vi "Validate_Cal_Date.vi"(10 "Calibration Limit(Days)":u32=120, 11 "Calibration File Paths":path[](array[path])=[path "C:/Users/Public/Documents/TDS Data/Rampage 5G HPA Pallet/Calibration/SigGen_plus_Cable.ini", path "C:/Users/Public/Documents/TDS Data/Rampage 5G HPA Pallet/Calibration/RF_to_UUT_HPA.ini", path "C:/Users/Public/Documents/TDS Data/Rampage 5G HPA Pallet/Calibration/RF_from_UUT_HPA.ini"]) -> (0 "Read Error?":bool, 1 "Calibration Due?":bool, 2 "found?":bool)   [LabVIEW 2025]
uses:
  <vilib>/Utility/miscctls.llb/LVDateTimeRec.ctl
  <vilib>/Utility/config.llb/Read Key (String).vi
  <vilib>/Utility/config.llb/NI_LVConfig.lvlib
panel:
  out "Current time":timestamp
  out "Calibration Date/Time":timestamp
  out "value":string
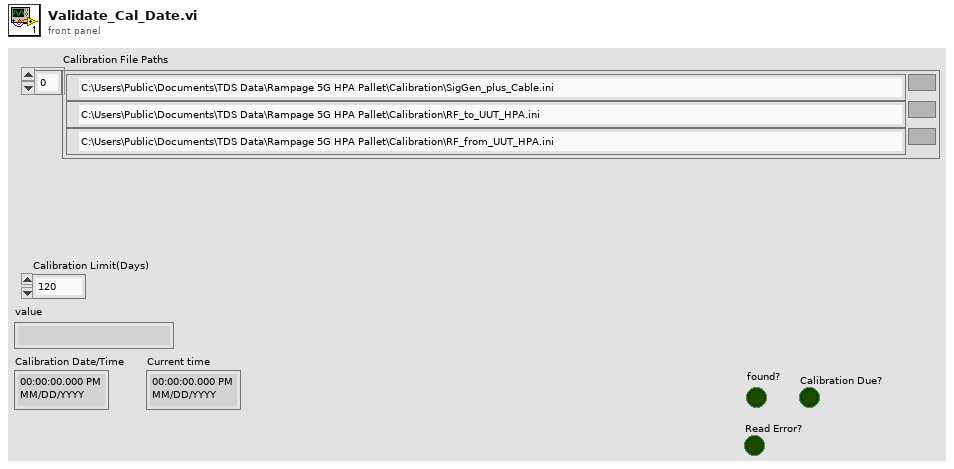
[diagram p1: front panel]
types:
  T1 = typedef "LVDateTimeRec.ctl" = cluster{"fractional second":dbl, "second":i32, "minute":i32, "hour":i32, "day of month":i32, "month":i32, "year":i32, "day of week":i32, "day of year":i32, "DST":i32}
  T2 = typedef "NI_LVConfig.lvlib/Config Data RefNum.ctl" = refnum<k1>
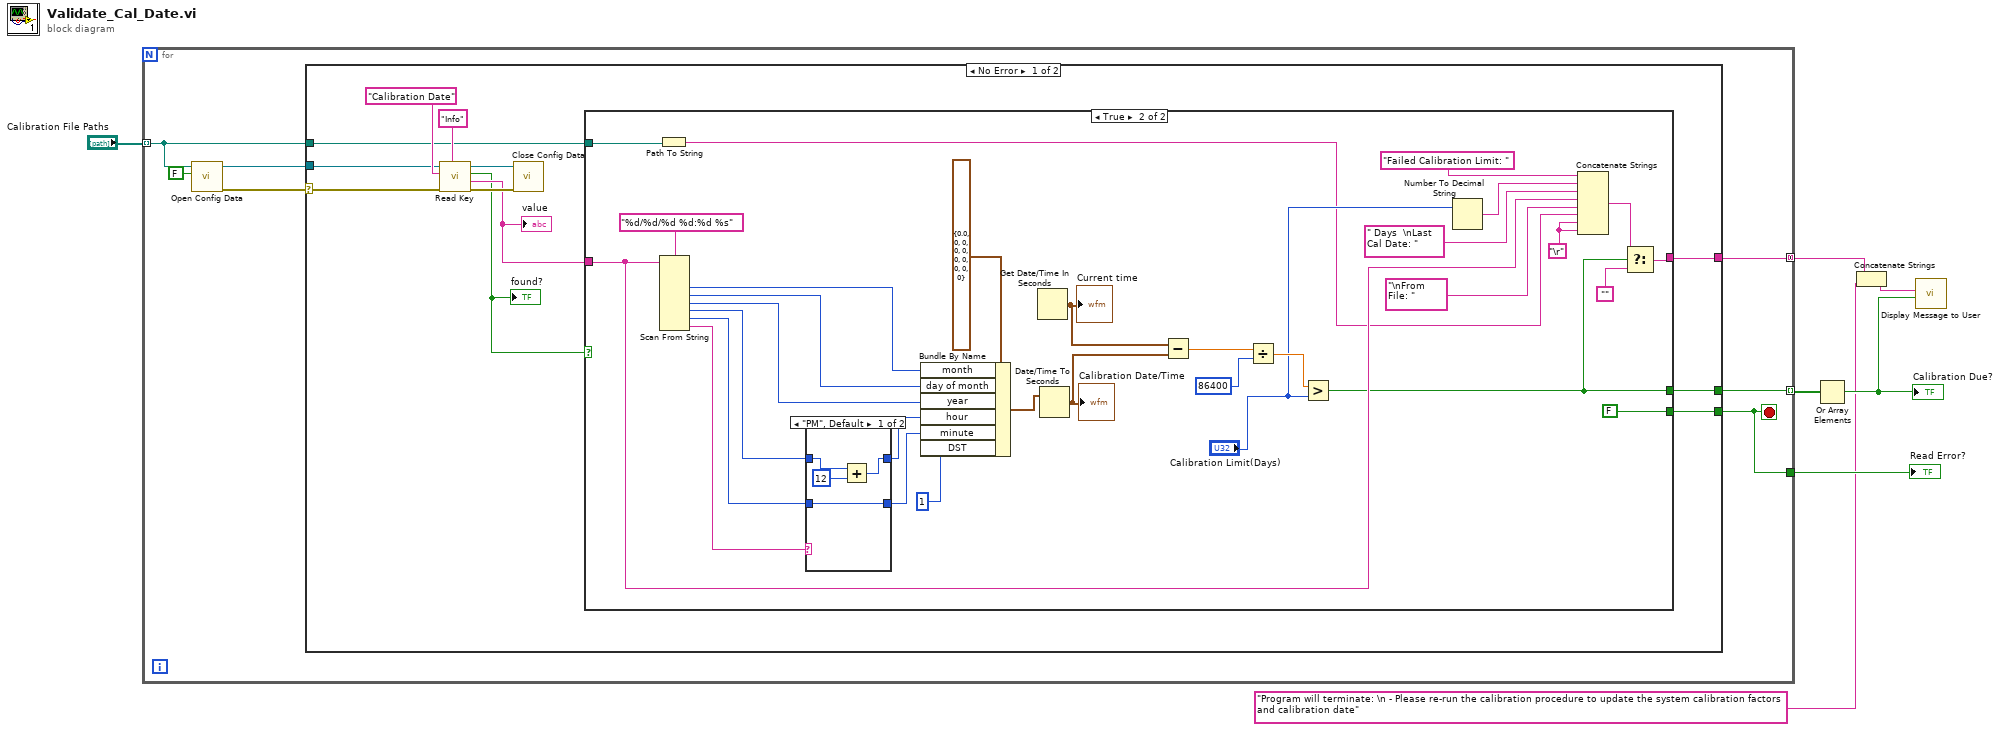
[diagram p0: block diagram]
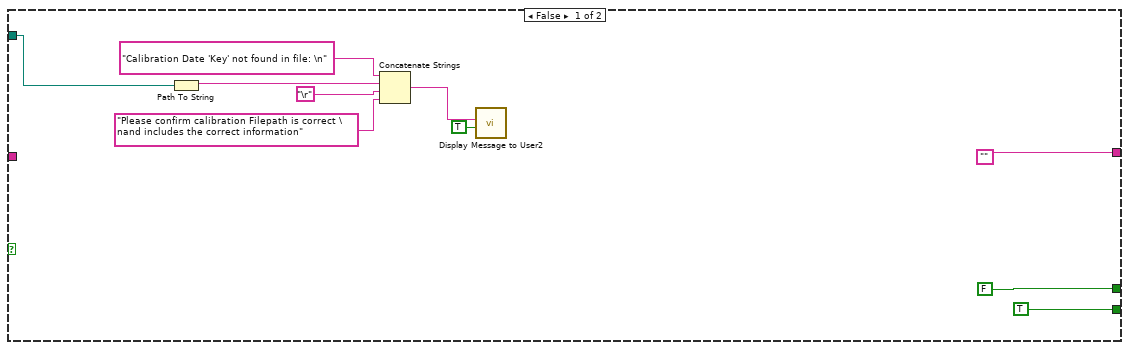
[diagram p2: hidden frame]
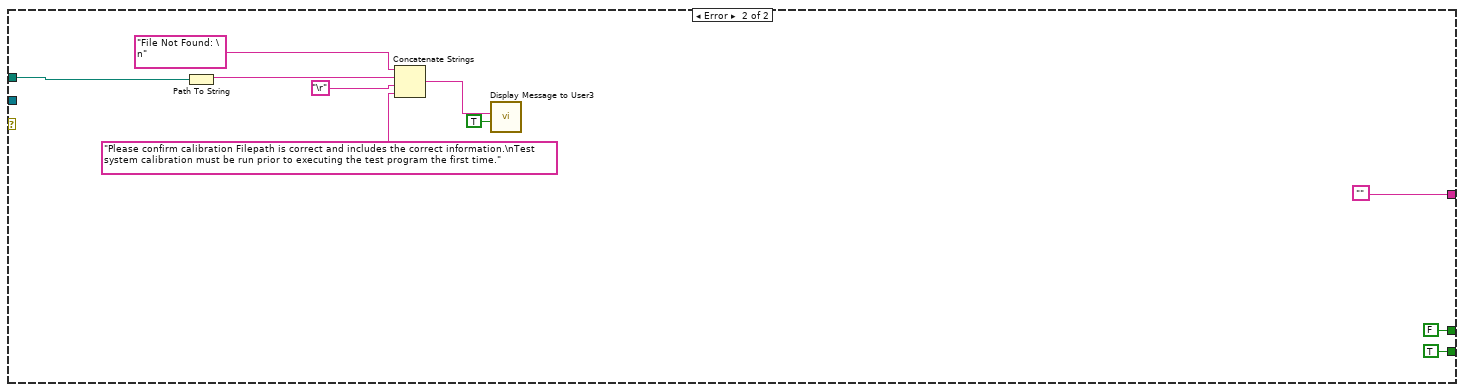
[diagram p4: hidden frame]
diagram:
  n1 = for {
    tunnel: "Calibration File Paths" -> [w13] mode=indexing
    tunnel: [w12] -> w6 mode=indexing
    tunnel: [w11] -> w5
    tunnel: [w10] -> w2 mode=concatenating
    stop <- w11 stop-if-true
    n2 = call <vilib>:"Open Config Data.vi"("create file if necessary (T)"=FALSE, "configuration file path"=w13) -> ("error out"=w9:errorcluster, "refnum"=w14:T2)  [unwired: 7 in, 1 out]
    n3 = case shown="No Error" w9 {
      selector: w9 -> [w15 _]
      tunnel: w14 -> [w24 _]
      tunnel: w13 -> [w19 w77]
      tunnel: [w18 FALSE] -> w12
      tunnel: [w17 TRUE] -> w11
      tunnel: [w16 ""] -> w10
      frame No Error {
        n4 = call-poly <vilib>:"Read Key.vi"("section"="Info", "error in (no error)"=w15, "key"="Calibration Date", "refnum"=w24) -> ("error out"=w22:errorcluster, "value"=w21:string, "found?"=w20:bool, "refnum out"=w23:T2)  [unwired: 4 in]
        "value" <- w21
        "found?" <- w20
        n5 = call <vilib>:"Close Config Data.vi"("error in (no error)"=w22, "refnum"=w23) -> ()  [unwired: 8 in, 2 out]
        n6 = case shown="True" w20 {
          tunnel: w21 -> [_ w49]
          tunnel: [FALSE w40] -> w18
          tunnel: w19 -> [w36 w48]
          tunnel: [TRUE FALSE] -> w17
          tunnel: ["" w37] -> w16
          frame False {
            n7 = Path To String(path=w36) -> (string=w34:string)
            n8 = Concatenate Strings("Calibration Date 'Key' not found in file: \n", w34, "\r", "Please confirm calibration Filepath is correct \nand includes the correct information") -> (w30:string)
            n9 = call "Display Message to User2"("Enable"=TRUE, "Message"=w30) -> ()  [unwired: 8 in, 2 out]
          }
          frame True {
            w41 = "\r"
            n10 = Path To String(path=w48) -> (string=w47:string)
            n11 = Scan From String(format string="%d/%d/%d %d:%d %s", input string=w49) -> (output 1=w65:i32, output 2=w64:i32, output 3=w63:i32, output 4=w60:i32, output 5=w58:i32, output 6=w61:string)  [unwired: 8 in, 3 out]
            n12 = case shown="\"PM\", Default" w61 {
              tunnel: [w71 w73] -> w59
              tunnel: w60 -> [w70 w73]
              tunnel: w58 -> [w68 w72]
              tunnel: [w68 w72] -> w57
              frame "PM", Default {
                n13 = Add(x=w70, y=12) -> (x+y=w71:i32)
              }
              frame "AM" {
              }
            }
            n14 = Bundle By Name(cluster=T1 {"fractional second"=0.0, "second"=0, "minute"=0, "hour"=0, "day of month"=0, "month"=0, "year"=0, "day of week"=0, "day of year"=0, "DST"=0} ("date time rec"), "month"=w65, "day of month"=w64, "year"=w63, "hour"=w59, "minute"=w57, "DST"=1) -> (w62:T1)
            n15 = Get Date/Time In Seconds() -> (seconds since 1Jan1904=w55:timestamp)
            "Current time" <- w55
            n16 = Date/Time To Seconds(2:w62) -> (0:w54:timestamp)  [unwired: 1 in]
            "Calibration Date/Time" <- w54
            n17 = Subtract(x=w55, y=w54) -> (x-y=w53:dbl)
            n18 = Divide(x=w53, y=86400) -> (x/y=w51:dbl)
            n19 = Greater?(x=w51, y="Calibration Limit(Days)") -> (0:w40:bool)
            n20 = Number To Decimal String(number="Calibration Limit(Days)") -> (decimal integer string=w45:string)  [unwired: 1 in]
            n21 = Concatenate Strings("Failed Calibration Limit: ", w45, " Days  \nLast Cal Date: ", w49, "\nFrom File: ", w47, w41, w41) -> (w39:string)
            n22 = Select(t=w39, s=w40, f="") -> (s? t:f=w37:string)
          }
        }
      }
      frame Error {
        n23 = Path To String(path=w77) -> (string=w82:string)
        n24 = Concatenate Strings("File Not Found: \n", w82, "\r", "Please confirm calibration Filepath is correct and includes the correct information.\nTest system calibration must be run prior to executing the test program the first time.") -> (w78:string)
        n25 = call "Display Message to User3"("Enable"=TRUE, "Message"=w78) -> ()  [unwired: 8 in, 2 out]
      }
    }
  }
  "Read Error?" <- w5
  n26 = Or Array Elements(Boolean array=w6) -> (logical OR=w4:bool)
  "Calibration Due?" <- w4
  n27 = Concatenate Strings(w2, "Program will terminate: \n - Please re-run the calibration procedure to update the system calibration factors and calibration date") -> (w3:string)
  n28 = call "Display Message to User"("Enable"=w4, "Message"=w3) -> ()  [unwired: 8 in, 2 out]
